vi "Get Click Location.vi"(8 "error in (no error)":errorcluster, 9 "Coords":T1, 10 "Tree Refnum":refnum<vi>, 11 "Test Executive Click Interpreter in":refnum<class "Test Executive Click Interpreter.lvclass">) -> (0 "error out":errorcluster, 1 "Valid?":bool, 2 "Insertion Index":i32, 3 "Parent ID":string, 5 "Tag":string)   [LabVIEW 2019, in "Test Executive Click Interpreter.lvclass"]
uses:
  <vilib>/gpm_packages/@cs/Test-executive-builder/Example/Application/Test Executive View/Test Executive Click Interpreter/Test Executive Click Interpreter.lvclass
  <vilib>/Utility/miscctls.llb/LVPoint32TypeDef.ctl
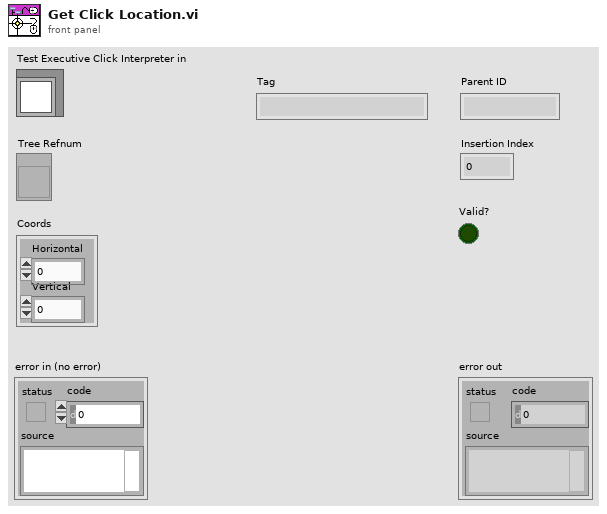
[diagram p1: front panel]
types:
  T1 = typedef "LVPoint32TypeDef.ctl" = cluster{"Horizontal":i32, "Vertical":i32}
  T2 = typedef "Relative Click Location.ctl" = enum16{"Unknown Location", "Below Element", "On Element", "Above Element"}
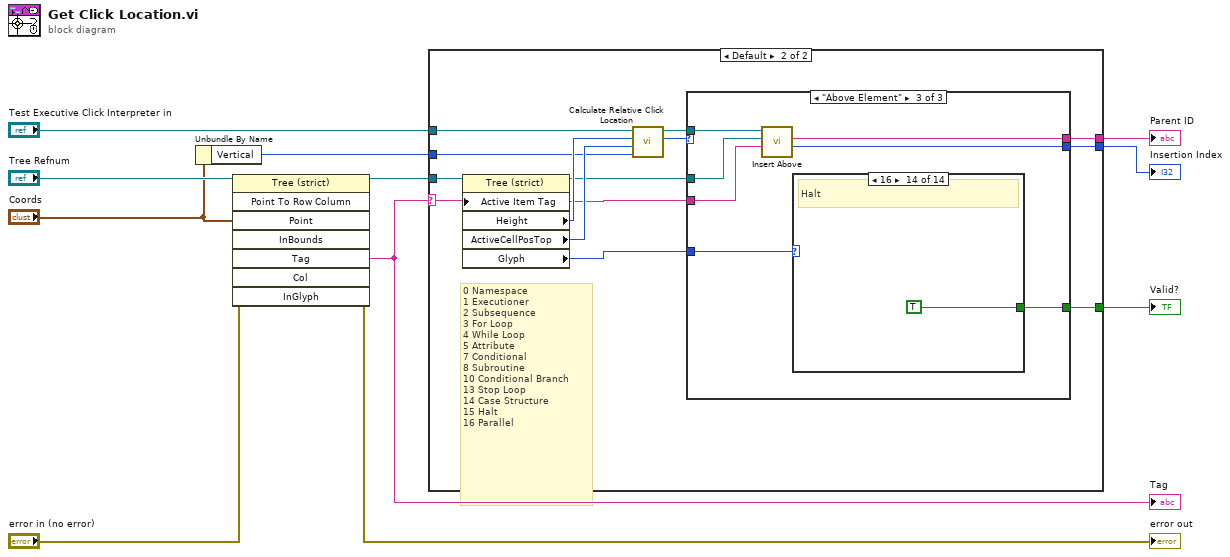
[diagram p0: block diagram]
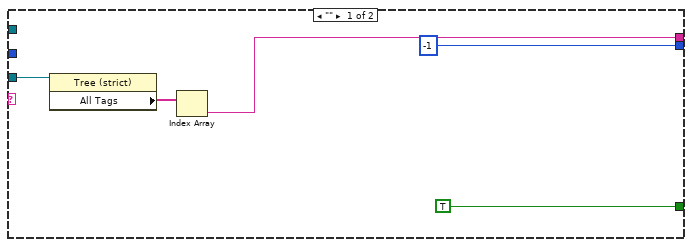
[diagram p2: hidden frame]
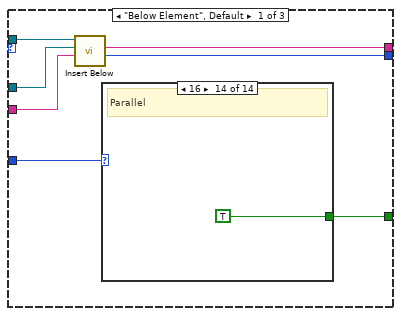
[diagram p3: hidden frame]
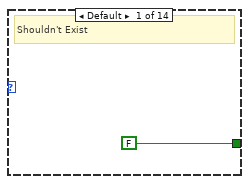
[diagram p4: hidden frame]
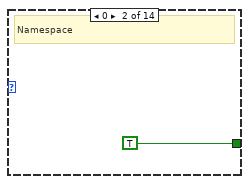
[diagram p5: hidden frame]
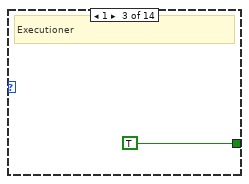
[diagram p6: hidden frame]
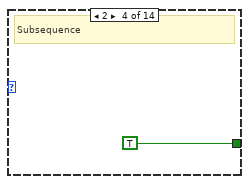
[diagram p7: hidden frame]
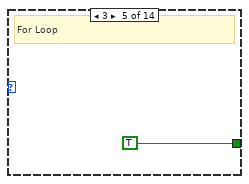
[diagram p8: hidden frame]
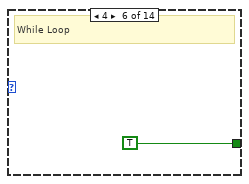
[diagram p9: hidden frame]
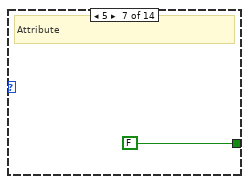
[diagram p10: hidden frame]
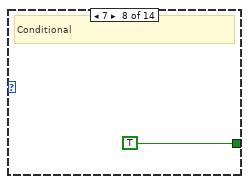
[diagram p11: hidden frame]
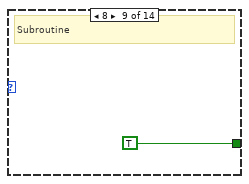
[diagram p12: hidden frame]
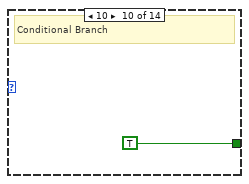
[diagram p13: hidden frame]
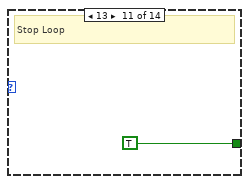
[diagram p14: hidden frame]
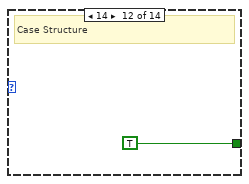
[diagram p15: hidden frame]
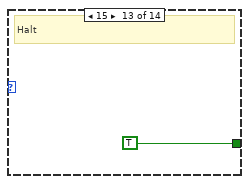
[diagram p16: hidden frame]
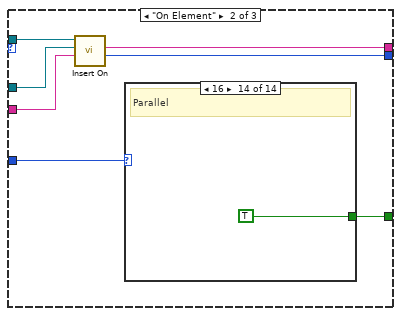
[diagram p17: hidden frame]
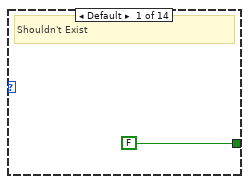
[diagram p18: hidden frame]
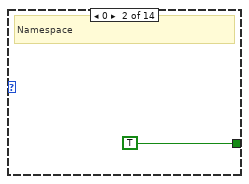
[diagram p19: hidden frame]
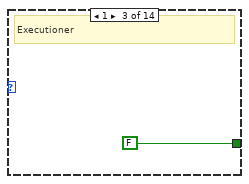
[diagram p20: hidden frame]
diagram:
  n1 = Unbundle By Name("Coords") -> ("Vertical"=w10:i32)
  n2 = invoke class="Tree (strict)" method="Point To Row Column"(reference="Tree Refnum", error in="error in (no error)", "Point"="Coords") -> (reference out=w11:refnum<vi>, error out=→"error out":errorcluster, "Tag"=w2:string)  [unwired: 5 in, 5 out]
  "Tag" <- w2
  n3 = case shown="Default" w2 {
    selector: w2 -> [_ w20]
    tunnel: [w14 w29] -> w4
    tunnel: [-1 ("Insertion Index") w28] -> w3
    tunnel: w11 -> [w16 w27]
    tunnel: "Test Executive Click Interpreter in" -> [_ w26]
    tunnel: w10 -> [_ w22]
    tunnel: [TRUE w17] -> w1
    frame "" {
      n4 = property class="Tree (strict)"(reference=w16) -> ("All Tags"=w15:string[])  [unwired: 1 in, 2 out]
      n5 = Index Array(array=w15) -> (element=w14:string)  [unwired: 1 in]
    }
    frame Default {
      # "0 Namespace\n1 Executioner\n2 Subsequence\n3 For Loop\n4 While Loop\n5 Attribute\n7 Conditional\n8 Subroutine\n10 Conditional Branch\n13 Stop Loop\n14 Case Structure\n15 Halt\n16 Parallel"
      n6 = property class="Tree (strict)"(reference=w27, "Active Item Tag"=w20) -> (reference out=w21:refnum<vi>, "Height"=w24:i32, "ActiveCellPosTop"=w23:i32, "Glyph"=w18:i32)  [unwired: 1 in, 1 out]
      n7 = call-dynamic "Calculate Relative Click Location.vi"("Click Vertical Position"=w22, "Cell Top Position"=w23, "Cell Height"=w24, "Tree Click Interpreter in"=w26) -> ("Relative Click Location"=w19:T2, "Tree Click Interpreter out"=w25:refnum<class "Test Executive Click Interpreter.lvclass">)  [unwired: 6 in]
      n8 = case shown="\"Above Element\"" w19 {
        tunnel: [w36 w54 w77] -> w29
        tunnel: [w35 w53 w76] -> w28
        tunnel: w25 -> [w34 w57 w78]
        tunnel: w21 -> [w33 w56 w75]
        tunnel: w20 -> [w32 w55 w74]
        tunnel: w18 -> [w31 w52 w73]
        tunnel: [w30 w51 w72] -> w17
        frame "Below Element", Default {
          n9 = call-dynamic "Insert Below.vi"("Item Tag"=w32, "Tree Refnum"=w33, "Tree Click Interpreter in"=w34) -> ("Insertion Index"=w35:i32, "Parent ID"=w36:string)  [unwired: 5 in, 2 out]
          n10 = case shown="16" w31 {
            tunnel: [FALSE TRUE TRUE TRUE TRUE TRUE FALSE TRUE TRUE TRUE TRUE TRUE TRUE TRUE] -> w30
            frame Default {
              # "Shouldn't Exist"
            }
            frame 0 {
              # "Namespace"
            }
            frame 1 {
              # "Executioner"
            }
            frame 2 {
              # "Subsequence"
            }
            frame 3 {
              # "For Loop"
            }
            frame 4 {
              # "While Loop"
            }
            frame 5 {
              # "Attribute"
            }
            frame 7 {
              # "Conditional"
            }
            frame 8 {
              # "Subroutine"
            }
            frame 10 {
              # "Conditional Branch"
            }
            frame 13 {
              # "Stop Loop"
            }
            frame 14 {
              # "Case Structure"
            }
            frame 15 {
              # "Halt"
            }
            frame 16 {
              # "Parallel"
            }
          }
        }
        frame "On Element" {
          n11 = call-dynamic "Insert On.vi"("Item Tag"=w55, "Tree Refnum"=w56, "Tree Click Interpreter in"=w57) -> ("Insertion Index"=w53:i32, "Parent ID"=w54:string)  [unwired: 5 in, 2 out]
          n12 = case shown="16" w52 {
            tunnel: [FALSE TRUE FALSE TRUE TRUE TRUE FALSE FALSE FALSE TRUE FALSE FALSE FALSE TRUE] -> w51
            frame Default {
              # "Shouldn't Exist"
            }
            frame 0 {
              # "Namespace"
            }
            frame 1 {
              # "Executioner"
            }
            frame 2 {
              # "Subsequence"
            }
            frame 3 {
              # "For Loop"
            }
            frame 4 {
              # "While Loop"
            }
            frame 5 {
              # "Attribute"
            }
            frame 7 {
              # "Conditional"
            }
            frame 8 {
              # "Subroutine"
            }
            frame 10 {
              # "Conditional Branch"
            }
            frame 13 {
              # "Stop Loop"
            }
            frame 14 {
              # "Case Structure"
            }
            frame 15 {
              # "Halt"
            }
            frame 16 {
              # "Parallel"
            }
          }
        }
        frame "Above Element" {
          n13 = call-dynamic "Insert Above.vi"("Item Tag"=w74, "Tree Refnum"=w75, "Tree Click Interpreter in"=w78) -> ("Insertion Index"=w76:i32, "Parent ID"=w77:string)  [unwired: 5 in, 2 out]
          n14 = case shown="16" w73 {
            tunnel: [FALSE TRUE TRUE TRUE TRUE TRUE FALSE TRUE TRUE TRUE TRUE TRUE TRUE TRUE] -> w72
            frame Default {
              # "Shouldn't Exist"
            }
            frame 0 {
              # "Namespace"
            }
            frame 1 {
              # "Executioner"
            }
            frame 2 {
              # "Subsequence"
            }
            frame 3 {
              # "For Loop"
            }
            frame 4 {
              # "While Loop"
            }
            frame 5 {
              # "Attribute"
            }
            frame 7 {
              # "Conditional"
            }
            frame 8 {
              # "Subroutine"
            }
            frame 10 {
              # "Conditional Branch"
            }
            frame 13 {
              # "Stop Loop"
            }
            frame 14 {
              # "Case Structure"
            }
            frame 15 {
              # "Halt"
            }
            frame 16 {
              # "Halt"
            }
          }
        }
      }
    }
  }
  "Parent ID" <- w4
  "Insertion Index" <- w3
  "Valid?" <- w1
